vi "write block diagram path constant.vi"(0 "VI Ref":refnum<vi>, 5 "constant path":path, 7 "constant label":string, 11 "error in":errorcluster) -> (4 "dup VI Ref":refnum<vi>, 15 "error out":errorcluster)   [LabVIEW 2020]
uses:
  <vilib>/Utility/traverseref.llb/TRef TravTarget.ctl
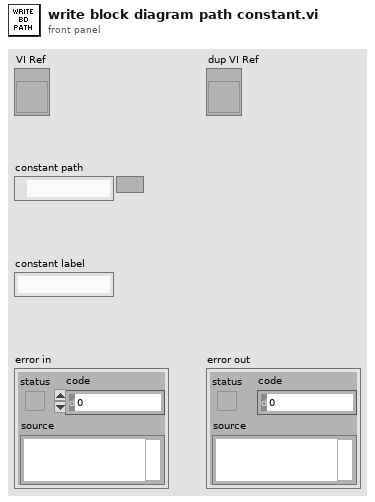
[diagram p1: front panel]
types:
  T1 = typedef "TRef TravTarget.ctl" = enum16{"FP", "BD", "Other"}
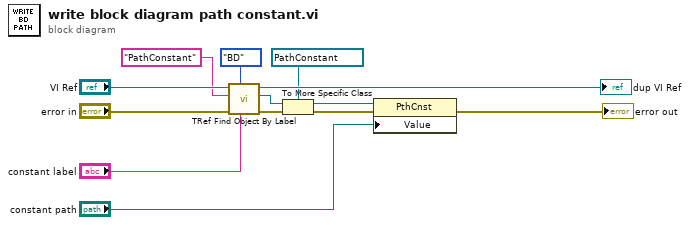
[diagram p0: block diagram]
diagram:
  n1 = call <vilib>:"TRef Find Object By Label.vi"("Label"="constant label", "Traverse Target"=TRef_TravTarget."BD", "error in (no error)"="error in", "Class Name"="PathConstant", "VI Ref"="VI Ref") -> ("error out"=w11:errorcluster, "Found Obj Ref"=w8:refnum<vi>, "dup VI Ref"=→"dup VI Ref":refnum<vi>)  [unwired: 3 in, 1 out]
  n2 = To More Specific Class(target class=refnum<vi> refnum ("Other Refnum"), reference=w8, error in=w11) -> (specific class reference=w9:refnum<vi>, error out=w12:errorcluster)
  n3 = property class="PthCnst"(reference=w9, error in=w12, "Value"="constant path") -> (error out=→"error out":errorcluster)  [unwired: 1 out]
